vi "UsrProfiles-Remove user.vi"   [LabVIEW 2017]
uses:
  Globals/gl_UsrProfiles globals.vi
types:
  T1 = typedef "User login window refs.ctl" = cluster{"User profiles window ref":refnum<k9>, "Users listbox":refnum<vi>, "Profiles listbox":refnum<vi>, "Last used":refnum<vi>}
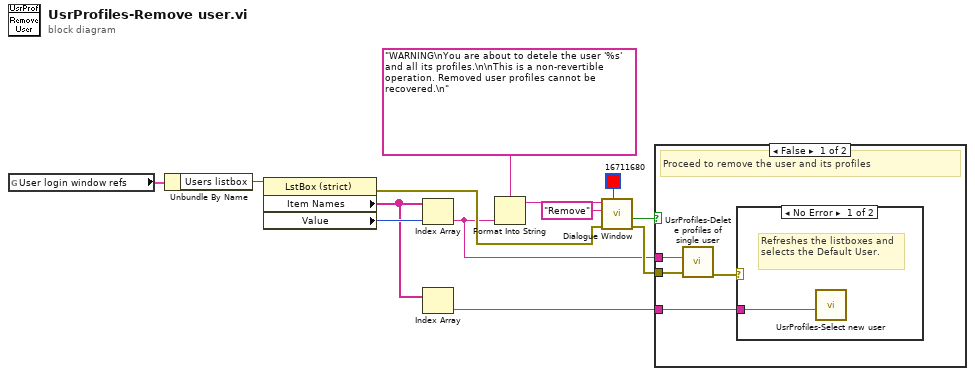
[diagram p0: block diagram]
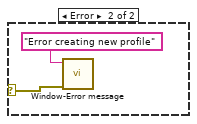
[diagram p2: hidden frame]
diagram:
  n1 = global read "gl_UsrProfiles globals.vi" "User login window refs"() -> (w11:T1)
  n2 = Unbundle By Name(w11) -> ("Users listbox"=w12:refnum<vi>)
  n3 = property on="Property Node" class="LstBox (strict)"(reference=w12) -> (error out=w6:errorcluster, "Item Names"=w4:string[], "Value"=w13:i32)  [unwired: 1 in, 1 out]
  n4 = Index Array(array=w4, index=w13) -> (element=w1:string)
  n5 = Index Array(array=w4) -> (element=w3:string)  [unwired: 1 in]
  n6 = Format Into String(format string="WARNING\nYou are about to detele the user '%s' and all its profiles.\n\nThis is a non-revertible operation. Removed user profiles cannot be recovered.\n" ("Message string"), w1) -> (resulting string=w9:string)  [unwired: 2 in, 1 out]
  n7 = call "Dialogue Window.vi"("Colour"=u32 16711680, "error in (no error)"=w6, "Caption-Right button (OK)"="Remove", "Message string"=w9) -> ("error out"=w5:errorcluster, "Cancelled (Left button pressed)"=w7:bool)  [unwired: 5 in, 1 out]
  n8 = case shown="False" w7 {
    tunnel: w5 -> [w16 _]
    tunnel: w3 -> [w17 _]
    tunnel: w1 -> [w14 _]
    frame False {
      # "Proceed to remove the user and its profiles"
      n9 = call "UsrProfiles-Delete profiles of single user.vi"("error in"=w16, "Name of user to remove"=w14) -> ("error out"=w15:errorcluster)  [unwired: 9 in]
      n10 = case shown="No Error" w15 {
        selector: w15 -> [_ w19]
        tunnel: w17 -> [w18 _]
        frame No Error {
          # "Refreshes the listboxes and selects the Default User."
          n11 = call "UsrProfiles-Select new user.vi"("New user name"=w18) -> ()  [unwired: 11 in]
        }
        frame Error {
          n12 = call "Window-Error message.vi"("error in (no error)"=w19, "Message"="Error creating new profile") -> ()  [unwired: 9 in, 1 out]
        }
      }
    }
    frame True {
      # "Cancelled"
    }
  }
